vi "GV DO6.vi"() -> ()   [LabVIEW 2017]
panel:
  out "DO6":bool
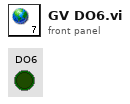
[diagram p1: front panel]
diagram:
